vi "GT Get Rand Code.vi"(8 "error in (no error)":errorcluster caption="错误输入（无错误）", 9 "pData":i16, 10 "addr":i16, 11 "cardNum":i16) -> (0 "error out":errorcluster caption="错误输出", 1 "pData out":i16, 3 "function return":i16)   [LabVIEW 2020, in "gts.lvlib"]
doc: "GT_API GT_GetRandCode(short cardNum,short addr,short *pData);"
uses:
  gts.lvlib
  dll/32bit/multi_card/gts.dll
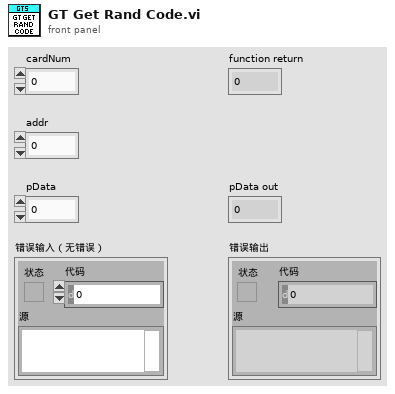
[diagram p1: front panel]
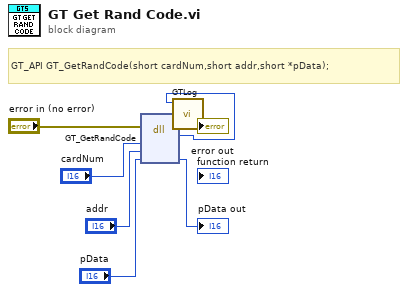
[diagram p0: block diagram]
diagram:
  # "GT_API GT_GetRandCode(short cardNum,short addr,short *pData);"
  n1 = dll-call lib="C:/1228/dll/32bit/multi_card/gts.dll" fn="GT_GetRandCode"(error in="error in (no error)", "cardNum"="cardNum", "addr"="addr", "pData"="pData") -> (error out=w3:errorcluster, w1:i16, "pData"=→"pData out":i16)  [unwired: 4 in, 1 out]
  n2 = call "GTLog.vi"("error in (no error)"=w3, "Numeric"=w1) -> ("error out"=→"error out":errorcluster)  [unwired: 9 in]
